vi "n_layer_nn_with_only_trained_params.vi"() -> ()   [LabVIEW 2020]
uses:
  Tanh.vi
  Sigmoid.vi
panel:
  in  "y":dbl[][](array[numeric])
  out "Sigmoid(Z)":dbl[][](array[numeric])
  in  "x":dbl[][](array[numeric])
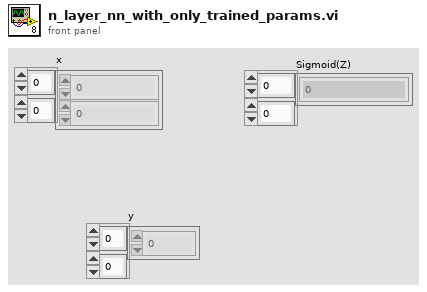
[diagram p1: front panel]
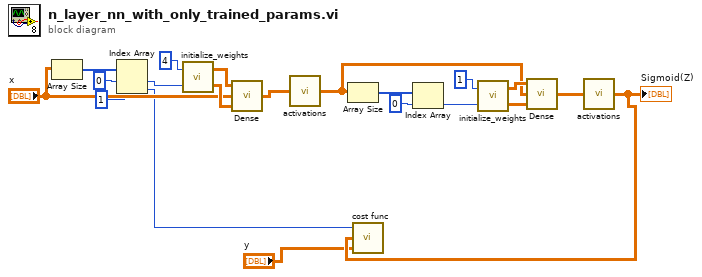
[diagram p0: block diagram]
diagram:
  n1 = Array Size(array="x") -> (size(s)=w19:i32[])
  n2 = Index Array(array=w19, index #1=0 ("index"), index #2=1 ("index")) -> (element #1=w17:i32, element #2=w3:i32)
  n3 = call "initialize_weights.vi"("n[l-1]"=w17, "n[l]"=4) -> ("b"=w15:dbl[][], "W"=w13:dbl[][])
  n4 = call "Dense.vi"("b"=w15, "A"="x", "w"=w13) -> ("Z"=w16:dbl[][])
  n5 = call-poly "activations.vi"("Z"=w16) -> ("Exp(Z)"=w8:dbl[][])  [unwired: 2 in]
  n6 = Array Size(array=w8) -> (size(s)=w9:i32[])
  n7 = Index Array(array=w9, index=0) -> (element=w6:i32)
  n8 = call "initialize_weights.vi"("n[l-1]"=w6, "n[l]"=1) -> ("b"=w11:dbl[][], "W"=w12:dbl[][])
  n9 = call "Dense.vi"("b"=w11, "A"=w8, "w"=w12) -> ("Z"=w5:dbl[][])
  n10 = call-poly "activations.vi"("Z"=w5) -> ("Sigmoid(Z)"=w2:dbl[][])  [unwired: 2 in]
  "Sigmoid(Z)" <- w2
  n11 = call "cost func.vi"("Y"="y", "A"=w2, "m"=w3) -> ()  [unwired: 1 out]
